vi "I2C_Data_hold_process.vi"(9 "waveform":waveform(dbl), 10 "VDDA":dbl=2.5, 11 "Index":dbl[](array[numeric])) -> (0 "Data ACK":bool, 1 "Data":u32=3999 format="%.0x", 2 "Address ACK":bool, 3 "Address":u32=2975 format="%.0x", 4 "Data Binary":bool[](array[boolean])=[TRUE, TRUE, TRUE, TRUE, TRUE, FALSE, FALSE, TRUE, TRUE, TRUE, TRUE, TRUE], 5 "Address Binary":bool[](array[boolean])=[TRUE, TRUE, TRUE, TRUE, TRUE, FALSE, FALSE, TRUE, TRUE, TRUE, FALSE, TRUE])   [LabVIEW 2019]
panel:
  out "Array 3":dbl[](array[numeric])=[0.03750000000000009, 2.4360937499999995, 0.05249999999999977, -0.05343750000000025, -0.017343750000000213, 2.4328125, 0.20250000000000012, 0.06046875000000007, -0.07593750000000021, 2.4351562499999995, 0.1846874999999999, -0.005156250000000195, 0.0885937499999998, -0.0070312500000002665, 0.5826562500000003, 2.338125, 2.4604687499999995, 0.04921875000000009, 0.05484374999999986, 0.03374999999999995, -0.01171875, 2.3404687499999994, 0.46734374999999995, 0.03937500000000016, 0.06796874999999991, 0.06000000000000005, 0.012187500000000018, 2.40046875, 0.1471874999999998, 0.029999999999999805, 0.03234374999999989, 0.00749999999999984, 0.7846874999999995, 2.4553125, -0.053906250000000266, 0.012187500000000018, -0.07828124999999986, 2.3390625, -0.014531250000000107, -0.08765625000000021, 0.03374999999999995, -0.030468750000000266, 0.08390625000000007, 2.44125, 0.1143749999999999, 0.039843749999999734, -0.020624999999999893, 0.04078124999999977, 0.06421874999999977, 0.07499999999999973, 0.6703124999999996, 2.3864062500000003, 2.32125, 2.39953125]
  out "size(s) 3":i32=13
  out "size(s) 2":i32=14
  out "subarray 2":dbl[](array[numeric])=[1.0, 1.0, 1.0, 1.0, 1.0, 0.0, 0.0, 1.0, 1.0, 1.0, 1.0, 1.0, 1.0]
  out "subarray":dbl[](array[numeric])=[1.0, 0.0, 1.0, 1.0, 1.0, 0.0, 0.0, 1.0, 1.0, 1.0, 1.0, 1.0, 1.0, 1.0]
  out "Clock pulses":i32=27
  out "size(s)":i32=56
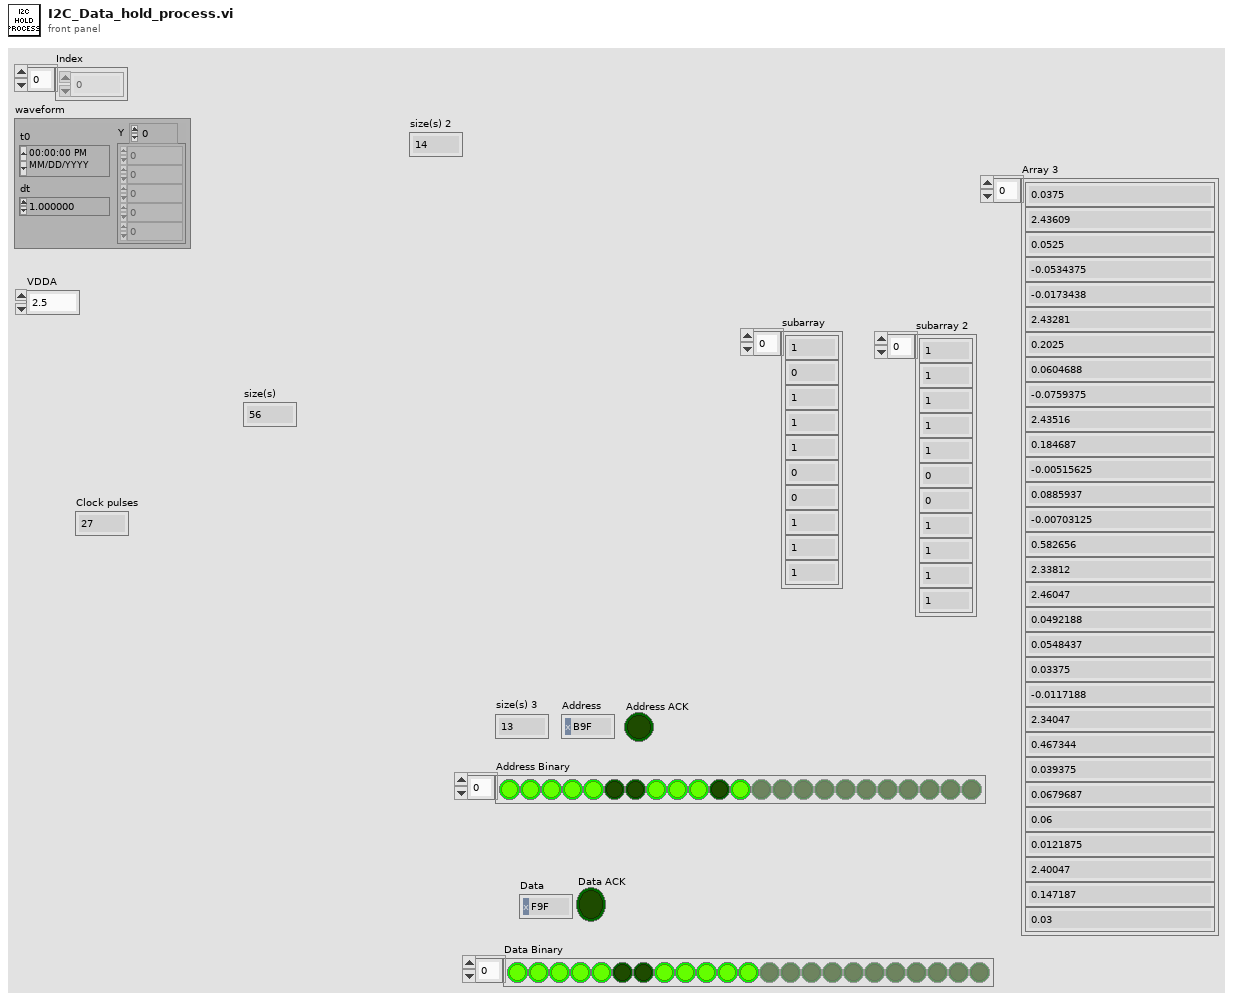
[diagram p1: front panel]
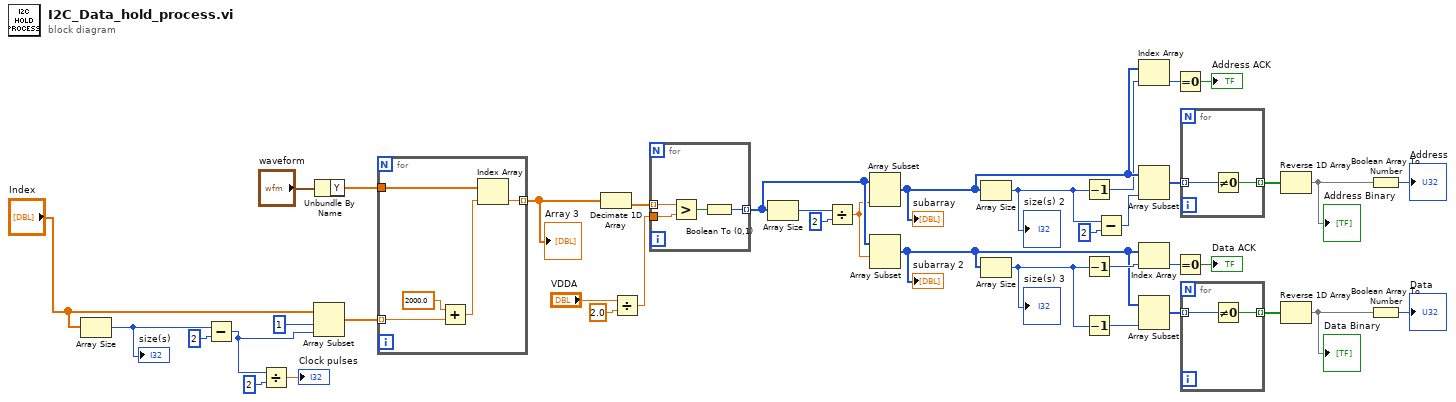
[diagram p0: block diagram]
diagram:
  n1 = Array Size(array="Index") -> (size(s)=w3:i32)
  "size(s)" <- w3
  n2 = Subtract(x=w3, y=2) -> (x-y=w33:i32)
  n3 = Divide(x=w33, y=2) -> (x/y=→"Clock pulses":dbl)
  n4 = Array Subset(array="Index", index=1, length=w33) -> (w37:dbl[])
  n5 = Unbundle By Name("waveform") -> ("Y"=w38:dbl[])
  n6 = for {
    tunnel: w37 -> [w44] mode=indexing
    tunnel: w38 -> [w45]
    tunnel: [w43] -> w34 mode=indexing
    n7 = Add(x=2000.0, y=w44) -> (x+y=w42:dbl)
    n8 = Index Array(array=w45, index=w42) -> (element=w43:dbl)
  }
  "Array 3" <- w34
  n9 = Decimate 1D Array(w34) -> (w30:dbl[])  [unwired: 1 out]
  n10 = Divide(x="VDDA", y=2.0) -> (x/y=w28:dbl)
  n11 = for {
    tunnel: w30 -> [w49] mode=indexing
    tunnel: w28 -> [w48]
    tunnel: [w46] -> w26 mode=indexing
    n12 = Greater?(x=w49, y=w48) -> (0:w47:bool)
    n13 = Boolean To (0,1)(Boolean=w47) -> (0, 1=w46:i16)
  }
  n14 = Array Size(array=w26) -> (size(s)=w32:i32)
  n15 = Divide(x=w32, y=2) -> (x/y=w25:dbl)
  n16 = Array Subset(array=w26, length=w25) -> (w21:i16[])  [unwired: 1 in]
  "subarray" <- w21
  n17 = Array Subset(array=w26, index=w25) -> (w9:i16[])  [unwired: 1 in]
  "subarray 2" <- w9
  n18 = Array Size(array=w21) -> (size(s)=w19:i32)
  "size(s) 2" <- w19
  n19 = Array Size(array=w9) -> (size(s)=w8:i32)
  "size(s) 3" <- w8
  n20 = Decrement(x=w19) -> (x-1=w17:i32)
  n21 = Decrement(x=w8) -> (x-1=w13:i32)
  n22 = Decrement(x=w8) -> (x-1=w7:i32)
  n23 = Subtract(x=w19, y=2) -> (x-y=w24:i32)
  n24 = Index Array(array=w21, index=w17) -> (element=w20:i16)
  n25 = Array Subset(array=w21, length=w24) -> (w23:i16[])  [unwired: 1 in]
  n26 = Index Array(array=w9, index=w13) -> (element=w12:i16)
  n27 = Array Subset(array=w9, length=w7) -> (w10:i16[])  [unwired: 1 in]
  n28 = Equal To 0?(x=w20) -> (x = 0?=→"Address ACK":bool)
  n29 = Equal To 0?(x=w12) -> (x = 0?=→"Data ACK":bool)
  n30 = for {
    tunnel: w23 -> [w51] mode=indexing
    tunnel: [w50] -> w15 mode=indexing
    n31 = Not Equal To 0?(x=w51) -> (x != 0?=w50:bool)
  }
  n32 = for {
    tunnel: w10 -> [w53] mode=indexing
    tunnel: [w52] -> w5 mode=indexing
    n33 = Not Equal To 0?(x=w53) -> (x != 0?=w52:bool)
  }
  n34 = Reverse 1D Array(array=w15) -> (reversed array=w6:bool[])
  "Address Binary" <- w6
  n35 = Reverse 1D Array(array=w5) -> (reversed array=w4:bool[])
  "Data Binary" <- w4
  n36 = Boolean Array To Number(Boolean array=w6) -> (number=→"Address":u32)
  n37 = Boolean Array To Number(Boolean array=w4) -> (number=→"Data":u32)
